vi "4Pi Cambridge Laser Routing.vi"(7 "Calling VI Ref":refnum<vi>) -> ()   [LabVIEW 2016]
uses:
  <vilib>/Utility/miscctls.llb/LVPointTypeDef.ctl
  <vilib>/ULx/Create Channel.llb/ULx Create Channel (DO-Digital Output).vi
  <vilib>/ULx/Write.llb/ULx Write (Digital Bool 1Line 1Point).vi
panel:
  in  "Quit":bool
  in  "Power Check":bool
  in  "4Pi":bool
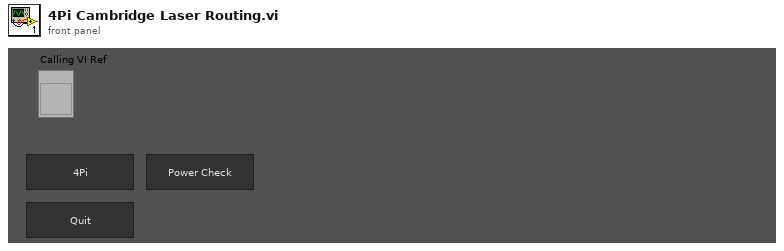
[diagram p1: front panel]
types:
  T1 = enum16{"Always On", "Always Off", "Off While Running"}
  T2 = typedef "LVPointTypeDef.ctl" = cluster{"Horizontal":i16, "Vertical":i16}
  T3 = typedef "LVRectTypeDef.ctl" = cluster{"Left":i16, "Top":i16, "Right":i16, "Bottom":i16}
  T4 = typedef "LVBoundsTypeDef.ctl" = cluster{"Width":u32, "Height":u32}
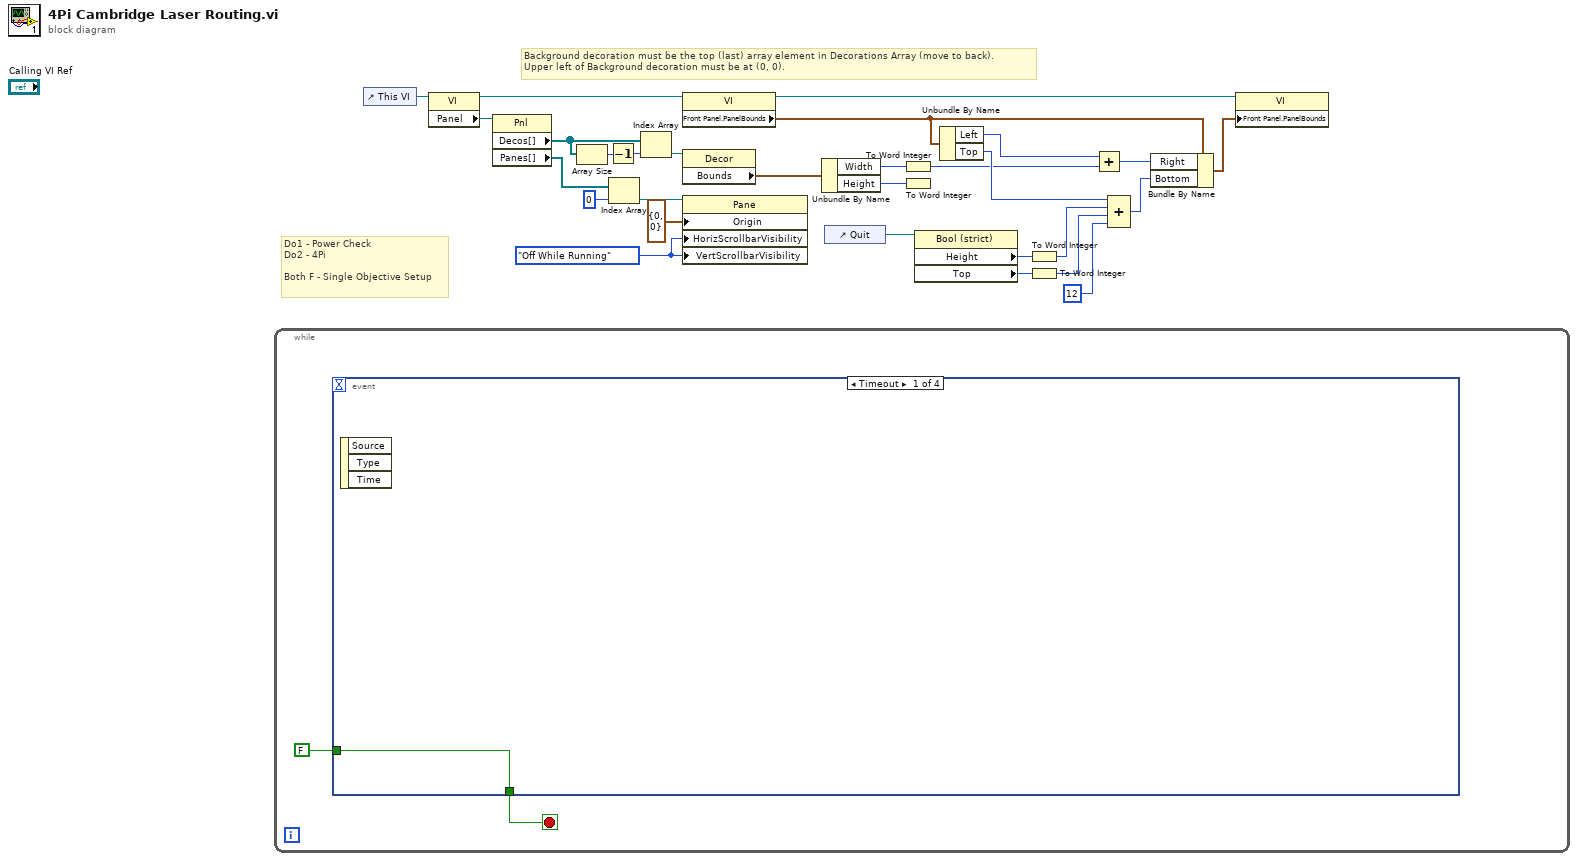
[diagram p0: block diagram]
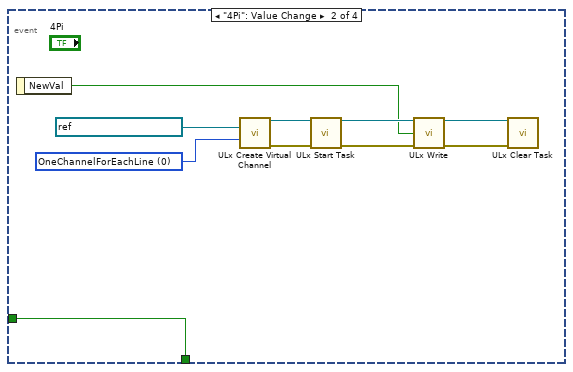
[diagram p2: hidden frame]
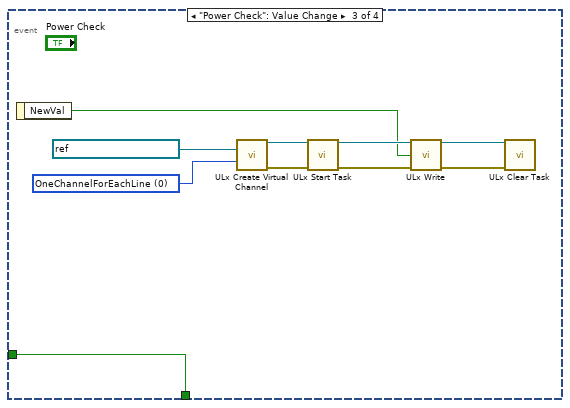
[diagram p3: hidden frame]
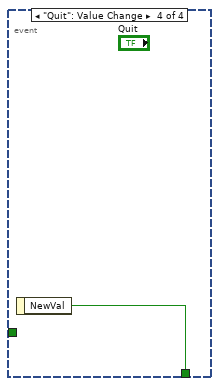
[diagram p4: hidden frame]
diagram:
  w12 = T1."Off While Running" ("Vertical Scrollbar Visibility")
  # "Background decoration must be the top (last) array element in Decorations Array (move to back).\nUpper left of Background decoration must be at (0, 0)."
  # "Do1 - Power Check\nDo2 - 4Pi\n\nBoth F - Single Objective Setup"
  n1 = while {
    stop <- w30 stop-if-true
    n2 = event shown="[0] Timeout" {
      selector: _ -> [_ _ _ _]
      dyn-events: _ -> [_ _ _ _]
      timeout: _ -> [_ _ _ _]
      tunnel: FALSE -> [w32 w34 w44 _]
      tunnel: [w32 w34 w44 w53] -> w30
      event Timeout {
        n3 = event-data() -> ()  [unwired: 1 in, 3 out]
      }
      event "4Pi": Value Change {
        w41 = 0 items=["OneChannelForEachLine", "OneChannelForAllLines"] ("line grouping")
        n4 = event-data() -> ("NewVal"=w33:bool)  [unwired: 1 in]
        n5 = call-poly <vilib>:"ULx Create Virtual Channel.vi"("lines"=refnum<k21> "Dev0/AuxPort/Do2", "line grouping"=w41) -> ("task out"=w40:refnum<k24>, "error out"=w39:errorcluster)  [unwired: 12 in]
        n6 = call <vilib>:"ULx Start Task.vi"("task in"=w40, "error in"=w39) -> ("task out"=w38:refnum<k24>, "error out"=w37:errorcluster)  [unwired: 12 in]
        n7 = call-poly <vilib>:"ULx Write.vi"("task in"=w38, "data"=w33, "error in"=w37) -> ("task out"=w36:refnum<k24>, "error out"=w35:errorcluster)  [unwired: 10 in, 1 out]
        n8 = call <vilib>:"ULx Clear Task.vi"("task in"=w36, "error in"=w35) -> ()  [unwired: 13 in, 1 out]
      }
      event "Power Check": Value Change {
        w51 = 0 items=["OneChannelForEachLine", "OneChannelForAllLines"] ("line grouping")
        n9 = event-data() -> ("NewVal"=w43:bool)  [unwired: 1 in]
        n10 = call-poly <vilib>:"ULx Create Virtual Channel.vi"("lines"=refnum<k21> "Dev0/AuxPort/Do2", "line grouping"=w51) -> ("task out"=w50:refnum<k24>, "error out"=w49:errorcluster)  [unwired: 12 in]
        n11 = call <vilib>:"ULx Start Task.vi"("task in"=w50, "error in"=w49) -> ("task out"=w48:refnum<k24>, "error out"=w47:errorcluster)  [unwired: 12 in]
        n12 = call-poly <vilib>:"ULx Write.vi"("task in"=w48, "data"=w43, "error in"=w47) -> ("task out"=w46:refnum<k24>, "error out"=w45:errorcluster)  [unwired: 10 in, 1 out]
        n13 = call <vilib>:"ULx Clear Task.vi"("task in"=w46, "error in"=w45) -> ()  [unwired: 13 in, 1 out]
      }
      event "Quit": Value Change {
        n14 = event-data() -> ("NewVal"=w53:bool)  [unwired: 1 in]
      }
    }
  }
  n15 = control-ref of="This VI"() -> (w4:refnum<vi>)
  n16 = property class="VI"(reference=w4) -> (reference out=w13:refnum<vi>, "Panel"=w5:refnum<vi>)  [unwired: 1 in, 1 out]
  n17 = property class="Pnl"(reference=w5) -> ("Decos[]"=w3:refnum<vi>[], "Panes[]"=w9:refnum<vi>[])  [unwired: 1 in, 2 out]
  n18 = Array Size(array=w3) -> (size(s)=w1:i32)
  n19 = Decrement(x=w1) -> (x-1=w2:i32)
  n20 = Index Array(array=w9, index=0) -> (element=w8:refnum<vi>)
  n21 = Index Array(array=w3, index=w2) -> (element=w11:refnum<vi>)
  n22 = property class="VI"(reference=w13) -> (reference out=w15:refnum<vi>, "Front Panel.PanelBounds"=w16:T3)  [unwired: 1 in, 1 out]
  n23 = property class="Decor"(reference=w11) -> ("Bounds"=w14:T4)  [unwired: 1 in, 2 out]
  n24 = property class="Pane"(reference=w8, "Origin"=T2 {"Horizontal"=0, "Vertical"=0}, "HorizScrollbarVisibility"=w12, "VertScrollbarVisibility"=w12) -> ()  [unwired: 1 in, 2 out]
  n25 = Unbundle By Name(w14) -> ("Width"=w19:u32, "Height"=w22:u32)
  n26 = control-ref of="Quit"() -> (w6:refnum<vi>)
  n27 = To Word Integer(number=w19) -> (16bit integer=w21:i16)
  n28 = To Word Integer(number=w22) -> ()  [unwired: 1 out]
  n29 = property class="Bool (strict)"(reference=w6) -> ("Height"=w24:u32, "Top"=w25:i32)  [unwired: 1 in, 2 out]
  n30 = Unbundle By Name(w16) -> ("Left"=w18:i16, "Top"=w29:i16)
  n31 = To Word Integer(number=w24) -> (16bit integer=w27:i16)
  n32 = To Word Integer(number=w25) -> (16bit integer=w28:i16)
  n33 = Add(x=w18, y=w21) -> (x+y=w20:i16)
  n34 = Compound Arithmetic op=ADD(w29, w27, w28, i16 12 ("y")) -> (w23:i16)
  n35 = Bundle By Name(cluster=w16, "Right"=w20, "Bottom"=w23) -> (w17:T3)
  n36 = property class="VI"(reference=w15, "Front Panel.PanelBounds"=w17) -> ()  [unwired: 1 in, 2 out]
